vi "Peg-in-hole 2015-03-09 a data.vi"() -> ()   [LabVIEW 2013]
uses:
  <vilib>/Analysis/baseanly.llb/Mean (DBL).vi
  <vilib>/Analysis/NI_AALBase.lvlib
  <vilib>/Analysis/NI_AALPro.lvlib
  <vilib>/gmath/NI_Gmath.lvlib
panel:
  in  "Times 2":dbl[](array[numeric])=[126.95, 36.6, 65.75, 57.35, 75.85, 36.85, 25.5, 26.1, 45.8, 158.25, 25.35, 15.7, 127.05, 98.35, 76.5, 46.15, 85.8, 57.7, 54.95, 47.9, 35.75, 47.35, 66.2, 15.35, 116.3, 26.45, 66.45, 16.0, 55.95, 26.9, 148.35, 47.152, 140.1, 16.201, 65.8, 15.45, 45.25, 36.95, 35.7, 15.75, 57.499, 15.75, 36.25, 122.1, 68.25, 203.25, 36.0, 68.1, 75.65, 88.2, 75.45, 99.4, 55.4, 108.6, 45.65, 99.1, 35.75, 173.4, 35.6, 89.5, 45.9, 183.05, 35.6, 110.95, 35.4, 129.85, 35.6, 67.4, 36.15, 77.05, 35.35, 171.55, 25.2, 78.45, 98.95, 15.2, 25.05, 170.75, 35.65, 67.3, 77.85, 66.65, 65.85, 130.9, 25.1, 110.35, 46.051, 15.15, 66.35, 297.45, 25.15, 150.4, 88.0, 113.1, 36.5, 90.75, 25.75, 143.35, 56.5, 78.4, 47.55, 310.05, 15.052, 77.5, 27.3, 67.6, 45.3, 15.35, 67.3, 36.45, 15.2, 87.95, 25.45, 233.9, 25.45, 76.75, 66.9, 108.85, 25.25, 15.85, 66.9, 141.05, 98.6, 15.75, 14.9, 26.15, 25.2, 56.2, 45.35, 15.45, 25.35, 35.8, 87.5, 15.25, 35.35, 15.55, 15.05, 15.4, 14.95, 77.6]
  in  "y":dbl
  out "correlation coefficient r":dbl
  out "offset":dbl
  out "power":dbl
  out "amplitude":dbl
  out "XY Graph":cluster{cluster{dbl, "mean":dbl}[]}[](graph)
  # "2 taught points"
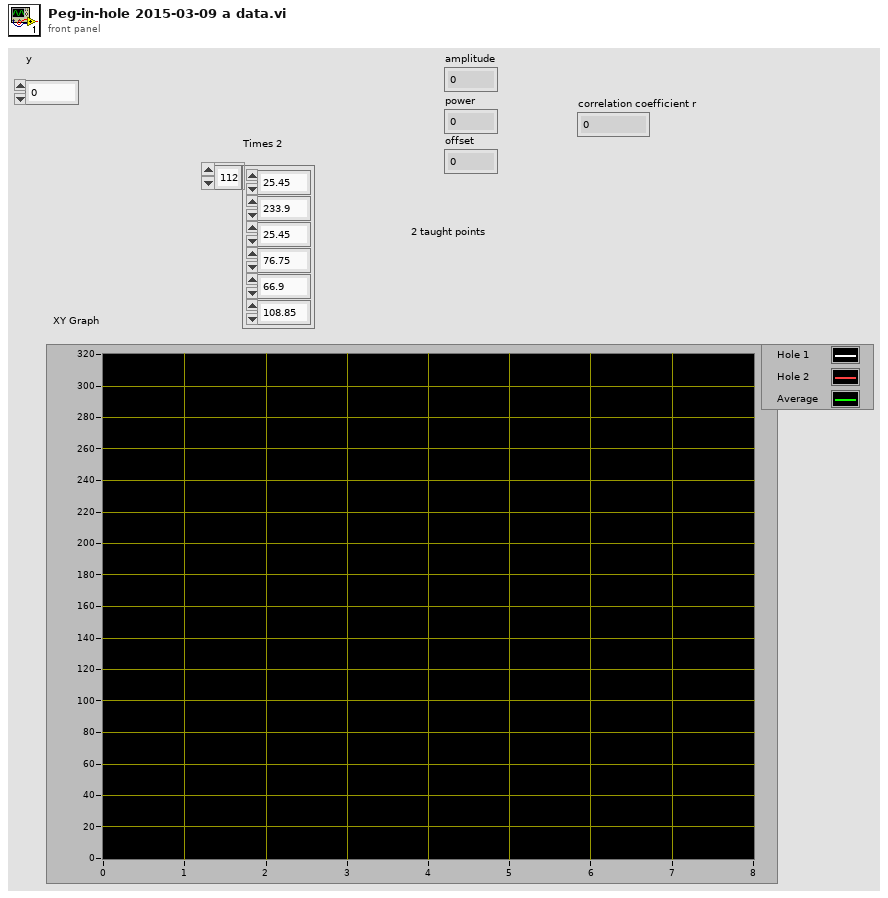
[diagram p1: front panel]
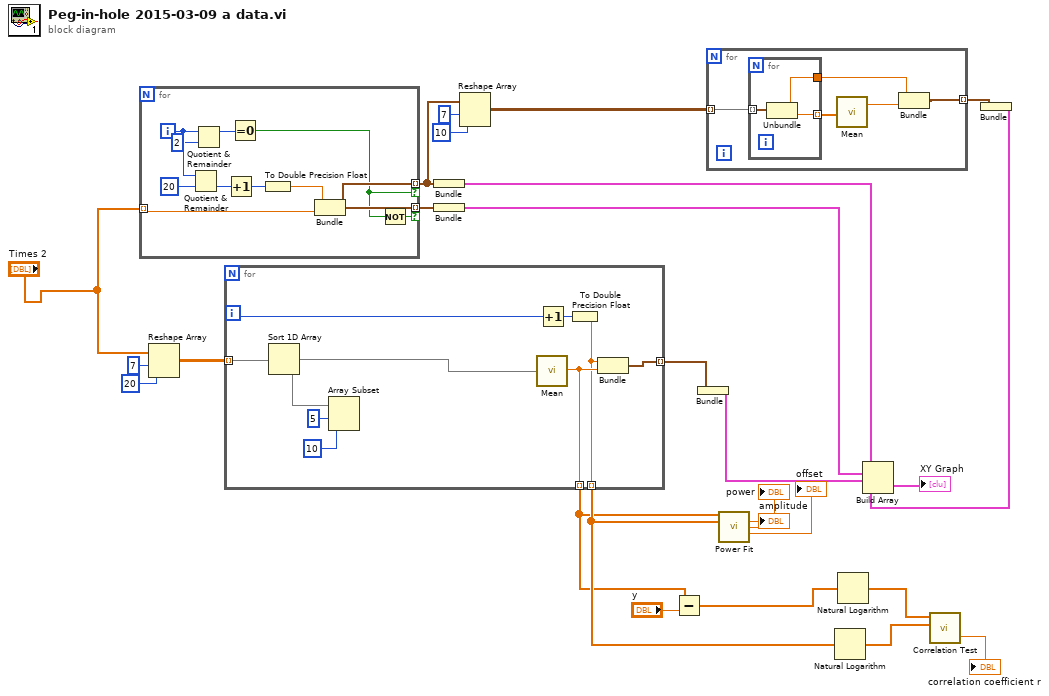
[diagram p0: block diagram]
diagram:
  n1 = for {
    tunnel: "Times 2" -> [w27] mode=indexing
    tunnel: [w30] -> w22 mode=indexing if=w28
    tunnel: [w30] -> w5 mode=indexing if=w29
    i -> [w33]
    n2 = Quotient & Remainder(x=w33, y=20) -> (floor(x/y)=w36:i32)  [unwired: 1 out]
    n3 = Quotient & Remainder(x=w33, y=2) -> (x-y*floor(x/y)=w31:i32)  [unwired: 1 out]
    n4 = Increment(x=w36) -> (x+1=w35:i32)
    n5 = Equal To 0?(x=w31) -> (x = 0?=w29:bool)
    n6 = To Double Precision Float(number=w35) -> (double precision float=w34:dbl)
    n7 = Bundle(w34, w27) -> (w30:cluster{dbl, dbl})  [unwired: 1 in]
    n8 = Not(x=w29) -> (.not. x?=w28:bool)
  }
  n9 = Reshape Array("Times 2", 7 ("dimension size"), 20 ("dimension size")) -> (w24:dbl[][])
  n10 = for {
    tunnel: w24 -> [w41] mode=indexing
    tunnel: [w44] -> w23 mode=indexing
    tunnel: [w43] -> w10 mode=indexing
    tunnel: [w42] -> w14 mode=indexing
    i -> [w46]
    n11 = Sort 1D Array(array=w41) -> (sorted array=w38:dbl[])
    n12 = Array Subset(array=w38, index=5, length=10) -> ()  [unwired: 1 out]
    n13 = call-poly <vilib>:"Mean.vi"("X"=w38) -> ("mean"=w43:dbl)  [unwired: 1 out]
    n14 = Increment(x=w46) -> (x+1=w45:i32)
    n15 = To Double Precision Float(number=w45) -> (double precision float=w42:dbl)
    n16 = Bundle(w42, "mean"=w43) -> (w44:cluster{dbl, "mean":dbl})  [unwired: 1 in]
  }
  n17 = Bundle(w5) -> (w8:cluster{cluster{dbl, dbl}[]})  [unwired: 1 in]
  n18 = Bundle(w22) -> (w20:cluster{cluster{dbl, dbl}[]})  [unwired: 1 in]
  n19 = Reshape Array(w5, 7 ("dimension size"), 10 ("dimension size")) -> (w4:cluster{dbl, dbl}[][])
  n20 = Subtract(x=w10, y="y") -> (x-y=w9:dbl[])
  n21 = Bundle(w23) -> (w19:cluster{cluster{dbl, "mean":dbl}[]})  [unwired: 1 in]
  n22 = for {
    tunnel: w4 -> [w51] mode=indexing
    tunnel: [w47] -> w3 mode=indexing
    n23 = for {
      tunnel: w51 -> [w54] mode=indexing
      tunnel: [w53] -> w50 mode=indexing
      tunnel: [w52] -> w49
      n24 = Unbundle(w54) -> (w52:dbl, w53:dbl)
    }
    n25 = call-poly <vilib>:"Mean.vi"("X"=w50) -> ("mean"=w48:dbl)  [unwired: 1 out]
    n26 = Bundle(w49, "mean"=w48) -> (w47:cluster{dbl, "mean":dbl})  [unwired: 1 in]
  }
  n27 = call <vilib>:"Power Fit.vi"("Y"=w10, "X"=w14) -> ("amplitude"=→"amplitude":dbl, "power"=→"power":dbl, "offset"=→"offset":dbl)  [unwired: 8 in, 3 out]
  n28 = Natural Logarithm(1:w14) -> (0:w12:dbl[])
  n29 = Natural Logarithm(1:w9) -> (0:w13:dbl[])
  n30 = call <vilib>:"Correlation Test.vi"("sample set y"=w12, "sample set x"=w13) -> ("correlation coefficient r"=→"correlation coefficient r":dbl)  [unwired: 5 in, 4 out]
  n31 = Bundle(w3) -> (w2:cluster{cluster{dbl, "mean":dbl}[]})  [unwired: 1 in]
  n32 = Build Array(w8, w20, w19, w2) -> (→"XY Graph":cluster{cluster{dbl, "mean":dbl}[]}[])
